vi "draw_pixmap.vi"(8 "error in":errorcluster, 11 "file_name":string="shell_volume.png") -> (0 "error out":errorcluster, 2 "status":bool, 3 "pict":picture, 4 "path":path)   [LabVIEW 2019]
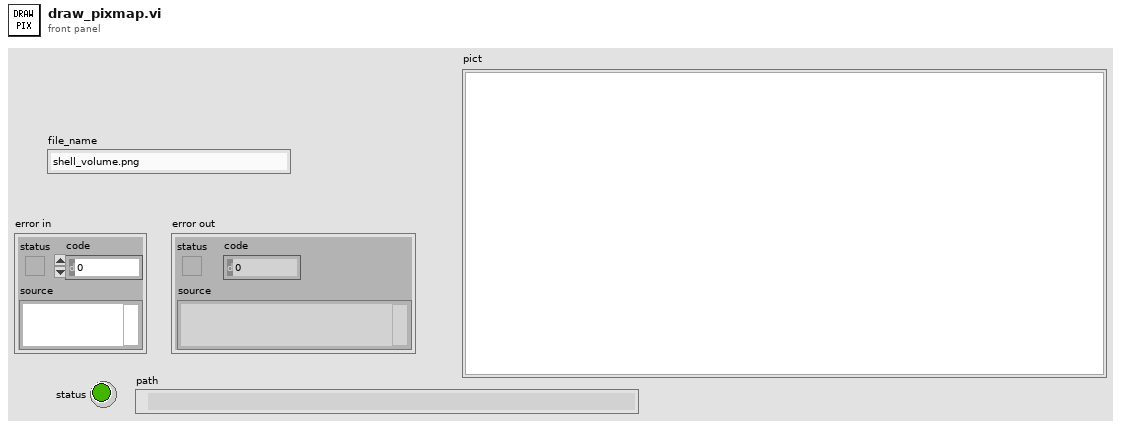
[diagram p1: front panel]
types:
  T1 = typedef "imagedata.ctl" = cluster{"image type":i32, "image depth":i32, "image":u8[], "mask":u8[], "colors":u32[], "Rectangle":cluster{"left":i16, "top":i16, "right":i16, "bottom":i16}}
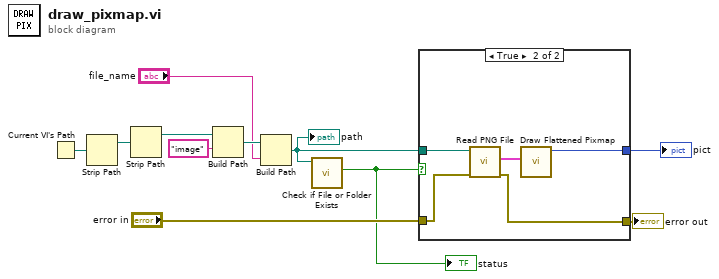
[diagram p0: block diagram]
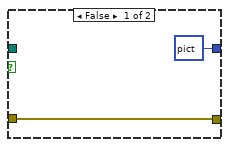
[diagram p2: hidden frame]
diagram:
  n1 = Current VI's Path() -> (path=w7:path)
  n2 = Strip Path(path=w7) -> (stripped path=w3:path)  [unwired: 1 out]
  n3 = Strip Path(path=w3) -> (stripped path=w2:path)  [unwired: 1 out]
  n4 = Build Path(base path=w2, name or relative path="image") -> (appended path=w5:path)
  n5 = Build Path(base path=w5, name or relative path="file_name") -> (appended path=w8:path)
  "path" <- w8
  n6 = call <vilib>:"Check if File or Folder Exists.vi"("path"=w8) -> ("file or folder exists?"=w9:bool)  [unwired: 8 in, 2 out]
  "status" <- w9
  n7 = case shown="True" w9 {
    tunnel: "error in" -> [w13 w17]
    tunnel: [w13 w14] -> w10
    tunnel: w8 -> [_ w18]
    tunnel: [picture data[5B] ("new picture") w15] -> w1
    frame False {
    }
    frame True {
      n8 = call <vilib>:"Read PNG File.vi"("error in (no error)"=w17, "path to PNG file"=w18) -> ("error out"=w14:errorcluster, "image data"=w16:T1)  [unwired: 7 in, 1 out]
      n9 = call <vilib>:"Draw Flattened Pixmap.vi"("image data"=w16) -> ("new picture"=w15:picture)  [unwired: 8 in]
    }
  }
  "error out" <- w10
  "pict" <- w1
